vi "Demo_Andon get max ID_OK.vi"(0 "Refnum in":T1, 5 "Station No.":string, 11 "error in (no error)":errorcluster) -> (4 "Refnum out":T1, 6 "MAX BREAKDOWN ID":i32, 8 "PRODUCTION COUNT":i32, 10 "TABLE NAME":string, 15 "error out":errorcluster)   [LabVIEW 2017]
uses:
  <vilib>/addons/database/Connection.llb/Conn ObjectReference.ctl
  <vilib>/addons/database/Connection.llb/Conn Execute.vi
  <vilib>/addons/database/Recordset.llb/Rec Fetch Recordset Data (R).vi
  <vilib>/addons/database/Recordset.llb/Rec Destroy - Connection.vi
  <vilib>/addons/database/NI_Database_API.lvlib
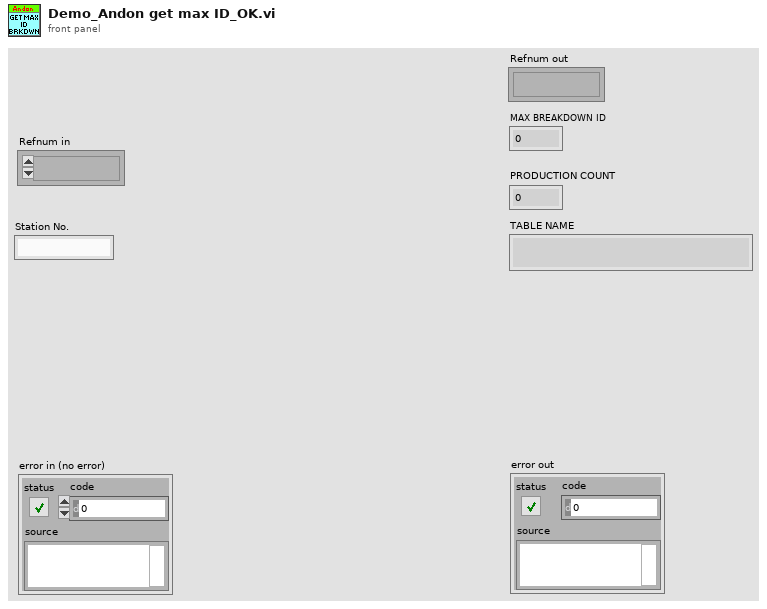
[diagram p1: front panel]
types:
  T1 = typedef "NI_Database_API.lvlib/Conn ObjectReference.ctl" = refnum<k1>
  T2 = typedef "NI_Database_API.lvlib/Rec ObjectReference.ctl" = refnum<k1>
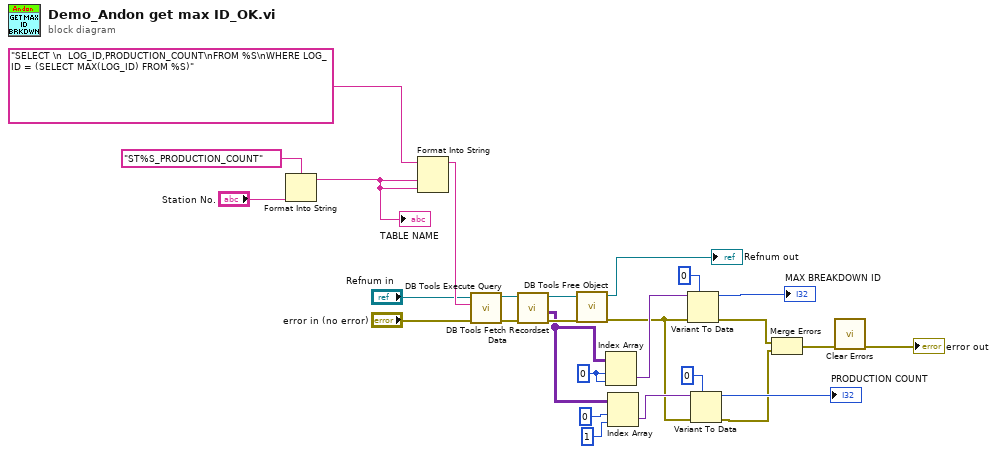
[diagram p0: block diagram]
diagram:
  w20 = 0 ("index (row)")
  n1 = Format Into String(format string="ST%S_PRODUCTION_COUNT" ("SQL query"), "Station No.") -> (resulting string=w15:string)  [unwired: 2 in, 1 out]
  "TABLE NAME" <- w15
  n2 = Format Into String(format string="SELECT \n  LOG_ID,PRODUCTION_COUNT\nFROM %S\nWHERE LOG_ID = (SELECT MAX(LOG_ID) FROM %S)" ("SQL query"), w15, w15) -> (resulting string=w19:string)  [unwired: 2 in, 1 out]
  n3 = call-poly <vilib>:"DB Tools Execute Query.vi"("error in (no error)"="error in (no error)", "SQL query"=w19, "connection reference"="Refnum in") -> ("error out"=w24:errorcluster, "recordset reference"=w25:T2)  [unwired: 5 in]
  n4 = call-poly <vilib>:"DB Tools Fetch Recordset Data.vi"("error in (no error)"=w24, "recordset reference"=w25) -> ("error out"=w23:errorcluster, "recordset data"=w11:variant[][], "recordset reference out"=w26:T2)  [unwired: 3 in]
  n5 = call-poly <vilib>:"DB Tools Free Object.vi"("error in (no error)"=w23, "recordset reference"=w26) -> ("error out"=w7:errorcluster, "connection reference"=→"Refnum out":T1)  [unwired: 8 in]
  n6 = Index Array(array=w11, index (row)=w20, index (col)=w20) -> (element=w21:variant)
  n7 = Index Array(array=w11, index (row)=0, index (col)=1) -> (element=w9:variant)
  n8 = Variant To Data(error in=w7, type=0, Variant=w21) -> (data=→"MAX BREAKDOWN ID":i32, error out=w3:errorcluster)
  n9 = Variant To Data(error in=w7, type=0, Variant=w9) -> (data=→"PRODUCTION COUNT":i32, error out=w4:errorcluster)
  n10 = Merge Errors(w3, w4) -> (w2:errorcluster)
  n11 = call <vilib>:"Clear Errors.vi"("error in (no error)"=w2) -> ("error out"=→"error out":errorcluster)  [unwired: 5 in, 1 out]
